vi "executemeasurement.vi"(0 "instrument handle in":refnum<k15>, 1 "Measurement Channel":T1(ring), 2 "Measurement  Selection":u16, 3 "Error In":errorcluster, 4 "Enabled Channels cluster":T2) -> (5 "Instrument handle out":refnum<k15>, 6 "result":dbl, 7 "Error Out":errorcluster)   [LabVIEW 2011]
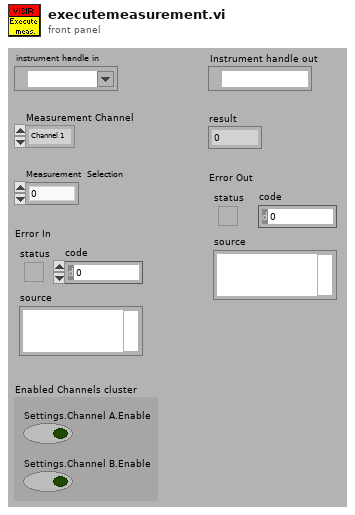
[diagram p1: front panel]
types:
  T1 = enum8{"Channel 1", "Channel 2", "Channel 3", "Channel 4"}
  T2 = cluster{"Settings.Channel A.Enable":bool, "Settings.Channel B.Enable":bool}
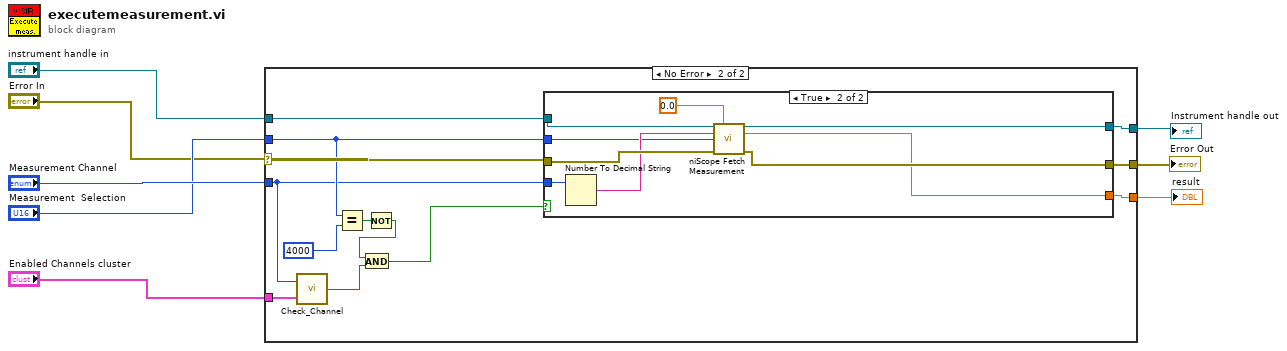
[diagram p0: block diagram]
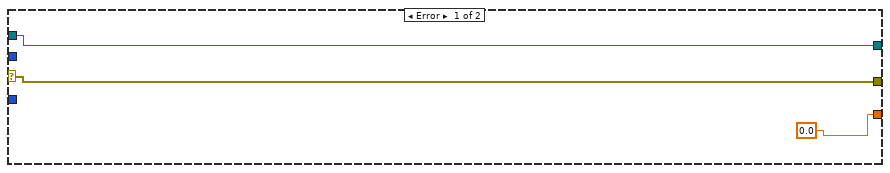
[diagram p2: hidden frame]
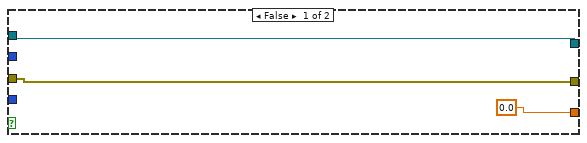
[diagram p3: hidden frame]
diagram:
  n1 = case shown="No Error" "Error In" {
    selector: "Error In" -> [w10 w20]
    tunnel: "Measurement Channel" -> [_ w13]
    tunnel: [0.0 w24] -> w7
    tunnel: [w10 w23] -> w6
    tunnel: [w9 w22] -> w5
    tunnel: "instrument handle in" -> [w9 w21]
    tunnel: "Measurement  Selection" -> [_ w15]
    tunnel: "Enabled Channels cluster" -> [_ w14]
    frame Error {
    }
    frame No Error {
      n2 = call "Check_Channel.vi"("Channels enabled"=w14, "Requested Channel"=w13) -> ("Boolean"=w18:bool)
      n3 = Equal?(x=w15, y=4000) -> (x = y?=w19:bool)
      n4 = Not(x=w19) -> (.not. x?=w12:bool)
      n5 = And(x=w12, y=w18) -> (x .and. y?=w16:bool)
      n6 = case shown="True" w16 {
        tunnel: w21 -> [w26 w36]
        tunnel: w20 -> [w27 w35]
        tunnel: w13 -> [_ w34]
        tunnel: w15 -> [_ w32]
        tunnel: [w26 w31] -> w22
        tunnel: [w27 w30] -> w23
        tunnel: [0.0 w29] -> w24
        frame False {
        }
        frame True {
          n7 = Number To Decimal String(number=w34) -> (decimal integer string=w33:string)  [unwired: 1 in]
          n8 = call <instrlib>:"niScope Fetch Measurement.vi"("instrument handle"=w36, "timeout"=0.0, "channels"=w33, "scalar measurement"=w32, "error in"=w35) -> ("instrument handle out"=w31:refnum<k15>, "result"=w29:dbl, "error out"=w30:errorcluster)  [unwired: 8 in]
        }
      }
    }
  }
  "result" <- w7
  "Error Out" <- w6
  "Instrument handle out" <- w5
